vi "niDDC Initialize.vi"(8 "error in (no error)":errorcluster, 9 "Option string":string, 10 "RIO0 Resource":T1 caption="RIO Device", 11 "Class in":refnum<class "7976R_v1.lvclass">) -> (0 "error out":errorcluster, 3 "Class out":refnum<class "7976R_v1.lvclass">)   [LabVIEW 2015, in "7976R_v1.lvclass"]
uses:
  <userlib>/SE-APP-Receiver/NI5772/7976R_v1/7976R_v1.lvclass
  <vilib>/userdefined/High Color/nirio_resource_hc.ctl
  <userlib>/SE-APP-Receiver/NI5772/7976R_v1/7976R_v1.lvclass/7976R_v1.ctl
  <vilib>/FPGAPlugInAG/PXIe-7976R/niLvFpga_Open_PXIe-7976R.vi
  <vilib>/rvi/interface/common/dynamic/niFpgaDynamicAddResources.vi
  <vilib>/FPGAPlugInAG/Dynamic/niLvFpga_Reset_Dynamic.vi
  <vilib>/FPGAPlugInAG/Dynamic/niLvFpga_Run_Dynamic.vi
  <vilib>/Utility/error.llb/Error Cluster From Error Code.vi
  <vilib>/rvi/errors/niLvFpgaAdjustHostInterfaceError.vi
  <vilib>/rvi/interface/nirviOpenFPGA/nirviOpenFPGA.xnode
  Users/Public/Documents/National Instruments/FPGA Extensions Bitfiles/NI PXIe-7976R/DDC with IDL v1.8_s7hk67NzjzY.lvbitx
  <vilib>/rvi/interface/nirviMethod/nirviMethod.xnode
  <vilib>/rvi/interface/nirviReadWriteControl/nirviReadWriteControl.xnode
  NiFpgaLv.dll
  <vilib>/rvi/interface/Simulation/niFpgaSimulationCallBeginRW.vi
panel:
  out "Fw Version":string
  out "Configured?":bool
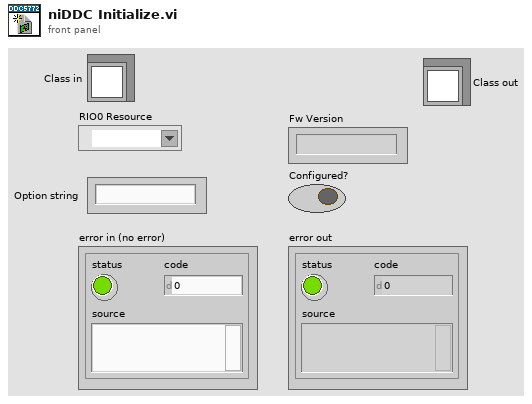
[diagram p1: front panel]
types:
  T1 = typedef "nirio_resource_hc.ctl" = tag
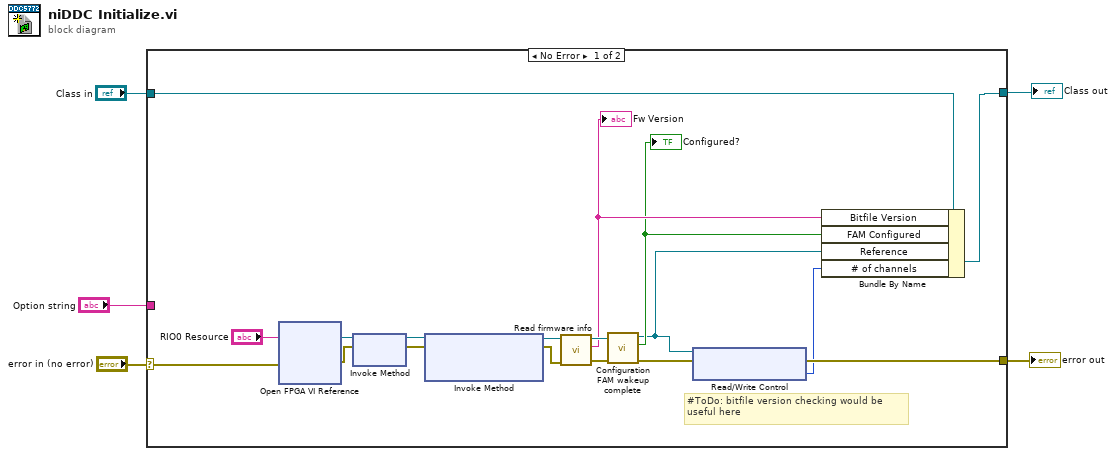
[diagram p0: block diagram]
diagram:
  n1 = case shown="No Error" "error in (no error)" {
    selector: "error in (no error)" -> [w14 w25]
    tunnel: [w8 w25] -> w5
    tunnel: "Class in" -> [w13 w24]
    tunnel: [w10 w24] -> w2
    tunnel: "Option string" -> [_ _]
    frame No Error {
      # "#ToDo: bitfile version checking would be \nuseful here"
      n2 = xnode "Open FPGA VI Reference"("error in"=w14, "resource name"="RIO0 Resource") -> ("FPGA VI Reference Out"=w21:refnum<k20>, "error out"=w22:errorcluster)
      n3 = xnode "Invoke Method"("FPGA VI Reference In"=w21, "error in"=w22) -> ("FPGA VI Reference Out"=w16:refnum<k20>, "error out"=w15:errorcluster)
      n4 = xnode "Invoke Method"("FPGA VI Reference In"=w16, "error in"=w15) -> ("FPGA VI Reference Out"=w17:refnum<k20>, "error out"=w18:errorcluster)  [unwired: 1 in]
      n5 = call <userlib>:"Read firmware info.vi"("error in (no error)"=w18, "Refnum in"=w17) -> ("error out"=w20:errorcluster, "Fw Version"=w12:string, "Refnum out"=w19:refnum<k20>)  [unwired: 7 in]
      "Fw Version" <- w12
      n6 = call <userlib>:"Configuration FAM wakeup complete.vi"("error in"=w20, "Ref in"=w19) -> ("error out"=w9:errorcluster, "Configured?"=w11:bool, "Ref out"=w6:refnum<k20>)  [unwired: 7 in]
      "Configured?" <- w11
      n7 = xnode "Read/Write Control"("FPGA VI Reference In"=w6, "error in"=w9) -> ("error out"=w8:errorcluster, "ddc.number.of.ch"=w7:u8)  [unwired: 1 out]
      n8 = Bundle By Name(cluster=w13, "Bitfile Version"=w12, "FAM Configured"=w11, "Reference"=w6, "# of channels"=w7) -> (w10:refnum<class "7976R_v1.lvclass">)
    }
    frame Error {
    }
  }
  "error out" <- w5
  "Class out" <- w2
